vi "Diagrams_coolprop.vi"(8 "error in (no error)":errorcluster, 9 "Path":path=path "C:/LABVIEW/LibFolder/CoolProp.dll", 10 "FluidOfInterest":T3="Water") -> (0 "error out":errorcluster, 1 "ph":cluster{dbl[], dbl[]}, 2 "Ts":cluster{dbl[], dbl[]}, 3 "Common Out":T1, 4 "Th":cluster{dbl[], dbl[]}, 5 "hs":cluster{dbl[], dbl[]}, 6 "pT":cluster{dbl[], dbl[]}, 7 "Fluid Data":T4)   [LabVIEW 2017]
doc: "Generates different arrays of fluid saturation points , which can be used to visualise different diagrams.\n\n---\nDesigned by Department of Industrial System and Product Design, Ghent University.\nContact: sergei.gusev@ugent.be; jan.nolens@ugent.be"
uses:
  FluidOfInterest.ctl
  FluidCommon.ctl
  FluidData.ctl
panel:
  out "Calculation":T1
  in  "Tab Control":T2(tab)
  out "Th diagram":cluster{dbl[], dbl[]}(graph)
  out "ph diagram":cluster{dbl[], dbl[]}(graph)
  out "Ts diagram":cluster{dbl[], dbl[]}(graph)
  out "hs diagram":cluster{dbl[], dbl[]}(graph)
  out "pT diagram":cluster{dbl[], dbl[]}(graph)
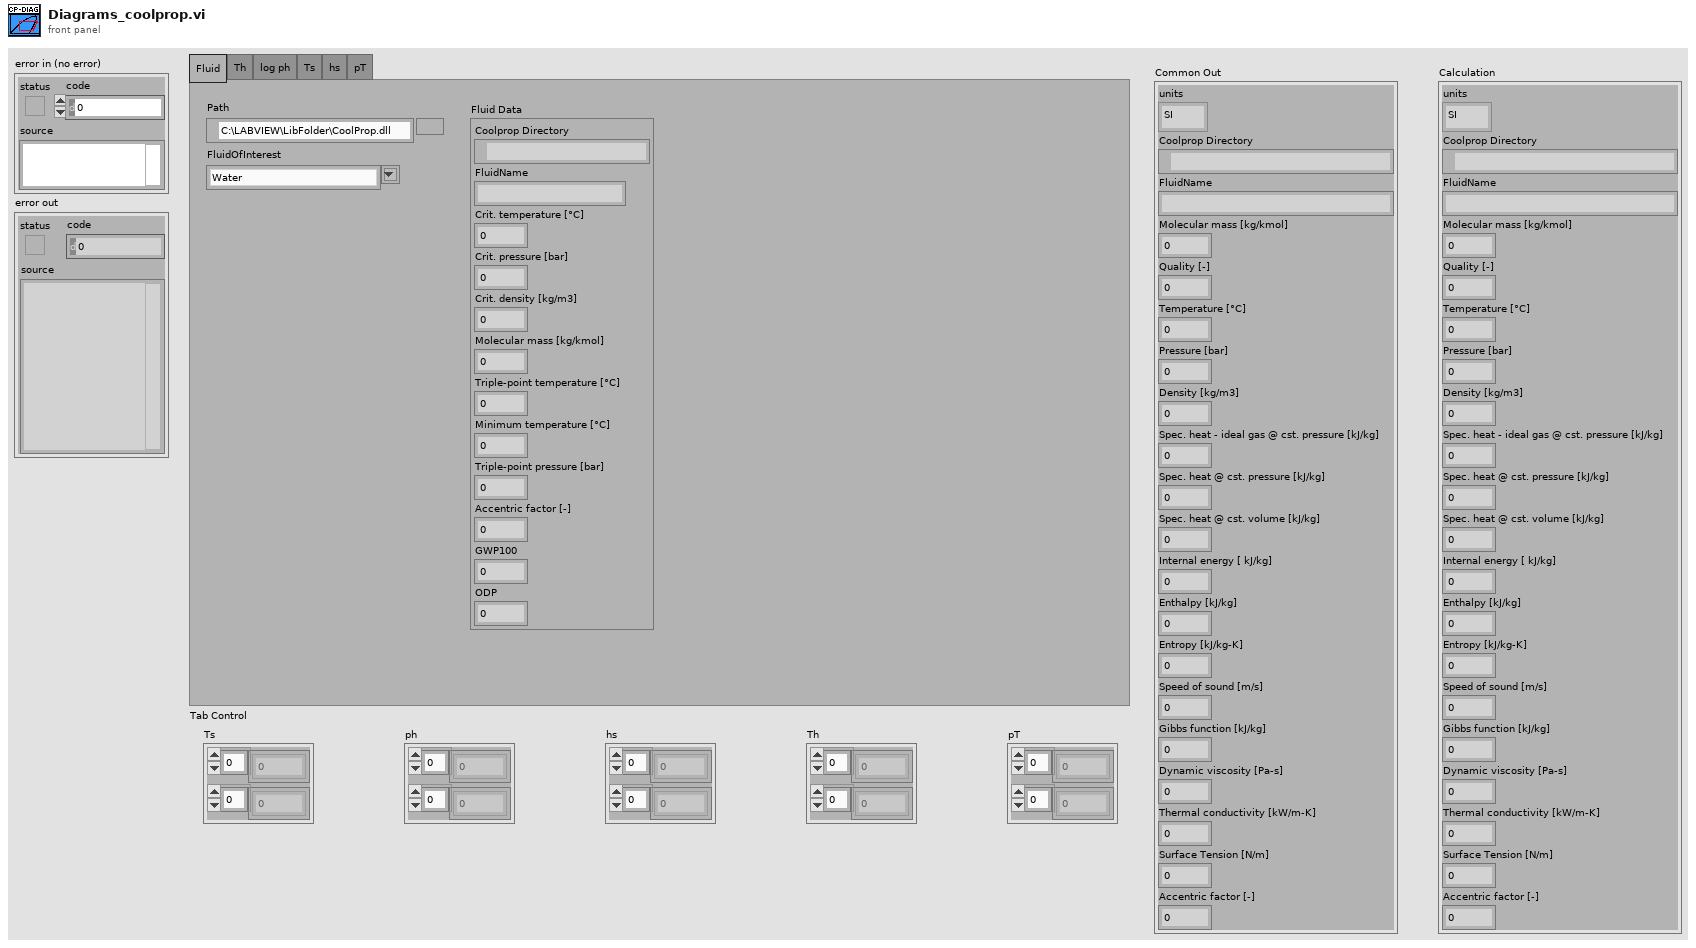
[diagram p1: front panel]
types:
  T1 = typedef "FluidCommon.ctl" = cluster{"units":enum16{"SI", "IP"}, "Coolprop Directory":path, "FluidName":string, "Molecular mass [kg/kmol]":dbl, "Quality [-]":dbl, "Temperature [°C]":dbl, "Pressure [bar]":dbl, "Density [kg/m3]":dbl, "Spec. heat - ideal gas @ cst. pressure [kJ/kg]":dbl, "Spec. heat @ cst. pressure [kJ/kg]":dbl, "Spec. heat @ cst. volume [kJ/kg]":dbl, "Internal energy [ kJ/kg]":dbl, "Enthalpy [kJ/kg]":dbl, "Entropy [kJ/kg-K]":dbl, "Speed of sound [m/s]":dbl, "Gibbs function [kJ/kg]":dbl, "Dynamic viscosity [Pa-s]":dbl, "Thermal conductivity [kW/m-K]":dbl, "Surface Tension [N/m]":dbl, "Accentric factor [-]":dbl}
  T2 = enum32{"Fluid", "Th", "log ph", "Ts", "hs", "pT"}
  T3 = typedef "FluidOfInterest.ctl" = string
  T4 = typedef "FluidData.ctl" = cluster{"Coolprop Directory":path, "FluidName":string, "Crit. temperature [°C]":dbl, "Crit. pressure [bar]":dbl, "Crit. density [kg/m3]":dbl, "Molecular mass [kg/kmol]":dbl, "Triple-point temperature [°C]":dbl, "Minimum temperature [°C]":dbl, "Triple-point pressure [bar]":dbl, "Accentric factor [-]":dbl, "GWP100":dbl, "ODP":dbl}
  T5 = enum16{"0", "TP", "TD", "PD", "TQ", "PQ", "HP", "SP", "SH"}
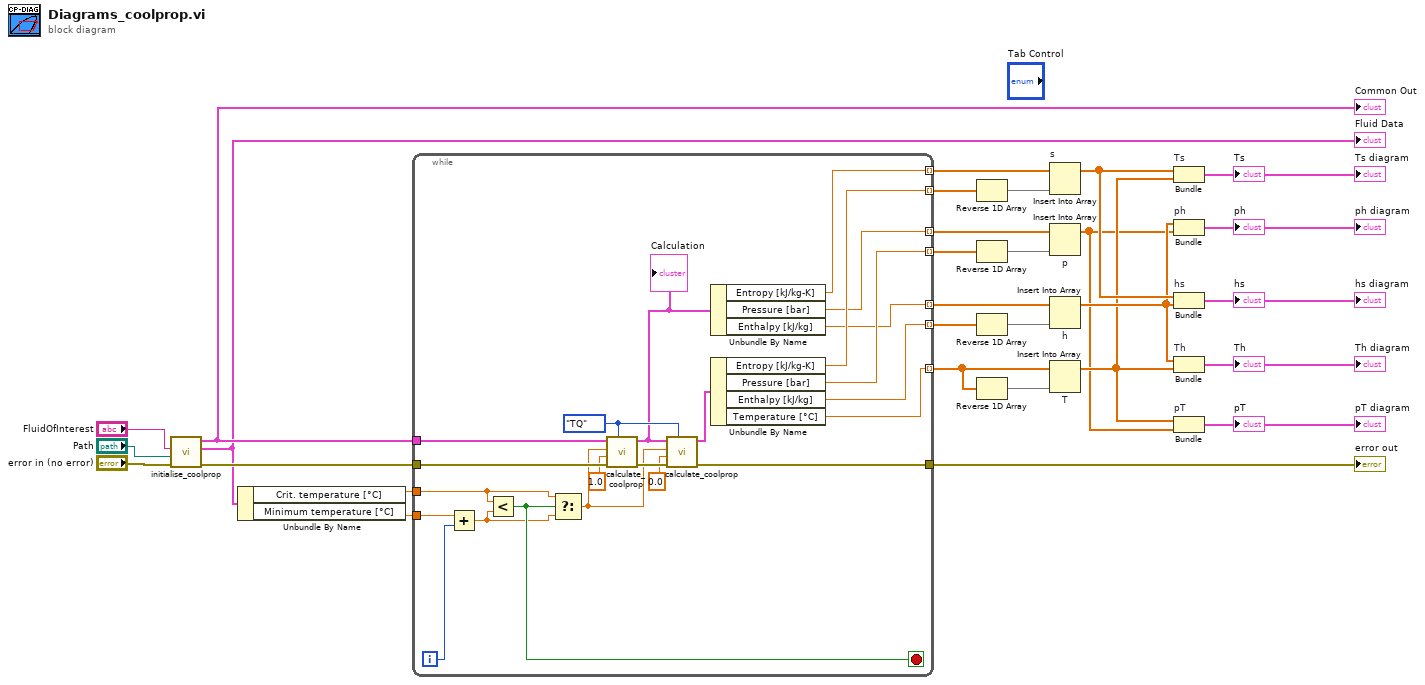
[diagram p0: block diagram]
diagram:
  n1 = call "initialise_coolprop.vi"("error in (no error)"="error in (no error)", "Path to CoolProp.dll"="Path", "FluidOfInterest"="FluidOfInterest") -> ("error out"=w17:errorcluster, "Fluid Data"=w15:T4, "Common Out"=w18:T1)  [unwired: 6 in]
  "Common Out" <- w18
  "Fluid Data" <- w15
  n2 = Unbundle By Name(w15) -> ("Crit. temperature [°C]"=w14:dbl, "Minimum temperature [°C]"=w13:dbl)
  n3 = while {
    tunnel: w18 -> [w51]
    tunnel: w17 -> [w50]
    tunnel: [w45] -> w16
    tunnel: w14 -> [w41]
    tunnel: w13 -> [w44]
    tunnel: [w33] -> w12 mode=indexing
    tunnel: [w30] -> w11 mode=indexing
    tunnel: [w31] -> w10 mode=indexing
    tunnel: [w34] -> w9 mode=indexing
    tunnel: [w35] -> w8 mode=indexing
    tunnel: [w32] -> w7 mode=indexing
    tunnel: [w36] -> w6 mode=indexing
    i -> [w43]
    stop <- w42 stop-if-true
    w48 = T5."TQ" ("InputCode")
    n4 = Add(x=w44, y=w43) -> (x+y=w40:dbl)
    n5 = Less?(x=w41, y=w40) -> (x < y?=w42:bool)
    n6 = Select(t=w41, s=w42, f=w40) -> (s? t:f=w39:dbl)
    n7 = call "calculate_coolprop.vi"("InputCode"=w48, "error in"=w50, "Input_2"=1.0, "Input_1"=w39, "Common In"=w51) -> ("error out"=w49:errorcluster, "Common Out"=w38:T1)  [unwired: 2 in]
    "Calculation" <- w38
    n8 = call "calculate_coolprop.vi"("InputCode"=w48, "error in"=w49, "Input_2"=0.0, "Input_1"=w39, "Common In"=w38) -> ("error out"=w45:errorcluster, "Common Out"=w37:T1)  [unwired: 2 in]
    n9 = Unbundle By Name(w38) -> ("Entropy [kJ/kg-K]"=w30:dbl, "Pressure [bar]"=w31:dbl, "Enthalpy [kJ/kg]"=w32:dbl)
    n10 = Unbundle By Name(w37) -> ("Entropy [kJ/kg-K]"=w33:dbl, "Pressure [bar]"=w34:dbl, "Enthalpy [kJ/kg]"=w35:dbl, "Temperature [°C]"=w36:dbl)
  }
  "error out" <- w16
  n11 = Reverse 1D Array(array=w12) -> (reversed array=w26:dbl[])
  n12 = Reverse 1D Array(array=w9) -> (reversed array=w27:dbl[])
  n13 = Reverse 1D Array(array=w8) -> (reversed array=w28:dbl[])
  n14 = Reverse 1D Array(array=w6) -> (reversed array=w29:dbl[])
  n15 = Insert Into Array "s"(array=w11, new element=w26) -> (w25:dbl[])  [unwired: 1 in]
  n16 = Insert Into Array "p"(array=w10, new element=w27) -> (w22:dbl[])  [unwired: 1 in]
  n17 = Insert Into Array "h"(array=w7, new element=w28) -> (w24:dbl[])  [unwired: 1 in]
  n18 = Insert Into Array "T"(array=w6, new element=w29) -> (w23:dbl[])  [unwired: 1 in]
  n19 = Bundle "Ts"(w25, w23) -> (→"Ts diagram" →"Ts":cluster{dbl[], dbl[]})  [unwired: 1 in]
  n20 = Bundle "ph"(w24, w22) -> (→"ph diagram" →"ph":cluster{dbl[], dbl[]})  [unwired: 1 in]
  n21 = Bundle "hs"(w25, w24) -> (→"hs diagram" →"hs":cluster{dbl[], dbl[]})  [unwired: 1 in]
  n22 = Bundle "Th"(w24, w23) -> (→"Th diagram" →"Th":cluster{dbl[], dbl[]})  [unwired: 1 in]
  n23 = Bundle "pT"(w23, w22) -> (→"pT diagram" →"pT":cluster{dbl[], dbl[]})  [unwired: 1 in]
